vi "agilent_measurement_test.vi"() -> ()   [LabVIEW 2016]
doc: "This VI shows how to do a logarithmic frequency sweep, and query the data from the PNA."
uses:
  <instrlib>/Keysight PNA Series/Keysight PNA Series.lvlib
panel:
  in  "Sweep Points (201)":i32=201
  out "Data":dbl[](graph)
  in  "Stop Frequency (1E+10 Hz)":dbl=6000000000.0
  in  "Start Frequency (1E+6 Hz)":dbl=1000000000.0
  in  "Measurement Name (MyMeas)":string="MyMeas"
  in  "Measurement Parameters (S22)":string="S22"
  in  "Channel (1)":i32=1
  in  "VISA resource name":refnum<visa-resource-name>="vna"
  # "(c) 2017 National Instruments.  ALL RIGHTS RESERVED."
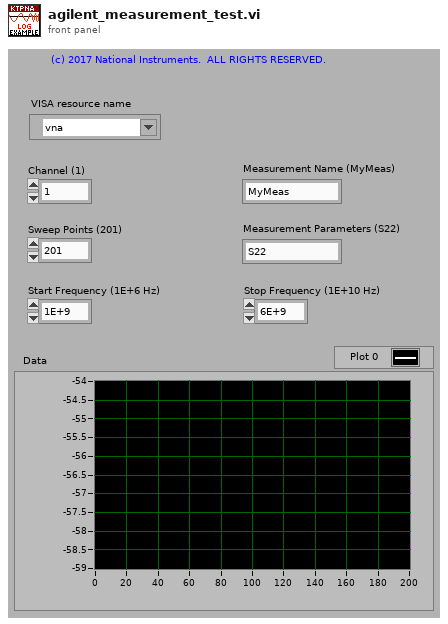
[diagram p1: front panel]
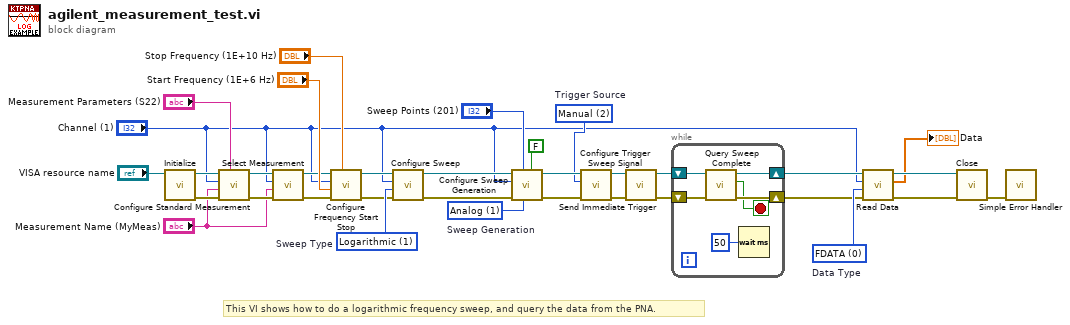
[diagram p0: block diagram]
diagram:
  w4 = 2 items=["Immediate", "External", "Manual"]  # Trigger Source
  w13 = 1 items=["Stepped", "Analog"]  # Sweep Generation
  w20 = 0 items=["FDATA", "RDATA", "SDATA", "FMEM", "SMEM", "SDIV"]  # Data Type
  w26 = 1 items=["Linear", "Logarithmic", "Power", "CW", "Segment", "Phase"]  # Sweep Type
  # "This VI shows how to do a logarithmic frequency sweep, and query the data from the PNA."
  n1 = call <instrlib>:"Initialize.vi"("VISA resource name"="VISA resource name") -> ("error out"=w32:errorcluster, "VISA resource name out"=w30:refnum<visa-resource-name>)  [unwired: 9 in]
  n2 = call <instrlib>:"Configure Standard Measurement.vi"("Measurement Parameters (S11)"="Measurement Parameters (S22)", "error in (no error)"=w32, "Measurement Name (CH1_S11_1)"="Measurement Name (MyMeas)", "Channel (1)"="Channel (1)", "VISA resource name"=w30) -> ("error out"=w31:errorcluster, "VISA resource name out"=w29:refnum<visa-resource-name>)  [unwired: 5 in]
  n3 = call <instrlib>:"Select Measurement.vi"("error in (no error)"=w31, "Measurement Name (CH1_S11_1)"="Measurement Name (MyMeas)", "Channel (1)"="Channel (1)", "VISA resource name"=w29) -> ("error out"=w10:errorcluster, "VISA resource name out"=w11:refnum<visa-resource-name>)  [unwired: 6 in]
  n4 = call <instrlib>:"Configure Frequency Start Stop.vi"("Stop Frequency (2E+6 Hz)"="Stop Frequency (1E+10 Hz)", "error in (no error)"=w10, "Start Frequency (1E+6 Hz)"="Start Frequency (1E+6 Hz)", "Channel (1)"="Channel (1)", "VISA resource name"=w11) -> ("error out"=w9:errorcluster, "VISA resource name out"=w12:refnum<visa-resource-name>)  [unwired: 5 in]
  n5 = call <instrlib>:"Configure Sweep.vi"("error in (no error)"=w9, "Sweep Type (0: Linear)"=w26, "Channel (1)"="Channel (1)", "VISA resource name"=w12) -> ("error out"=w19:errorcluster, "VISA resource name out"=w18:refnum<visa-resource-name>)  [unwired: 6 in]
  n6 = call <instrlib>:"Configure Sweep Generation.vi"("Auto Sweep or Dwell Time (T: Enable)"=FALSE ("Enable Auto Sweep/Dwell Time (T: Enable)"), "Sweep Generation (1: Analog)"=w13, "Sweep Points (201)"="Sweep Points (201)", "error in (no error)"=w19, "Channel (1)"="Channel (1)", "VISA resource name"=w18) -> ("error out"=w8:errorcluster, "VISA resource name out"=w6:refnum<visa-resource-name>)  [unwired: 4 in]
  n7 = call <instrlib>:"Configure Trigger Sweep Signal.vi"("error in (no error)"=w8, "Trigger Source (0: Immediate)"=w4, "VISA resource name"=w6) -> ("error out"=w3:errorcluster, "VISA resource name out"=w2:refnum<visa-resource-name>)  [unwired: 7 in]
  n8 = call <instrlib>:"Send Immediate Trigger.vi"("error in (no error)"=w3, "VISA resource name"=w2) -> ("error out"=w7:errorcluster, "VISA resource name out"=w5:refnum<visa-resource-name>)  [unwired: 8 in]
  n9 = while {
    shift-right: [w39] -> w15
    shift-left: w7 -> [w40]
    shift-right: [w36] -> w14
    shift-left: w5 -> [w37]
    stop <- w38 stop-if-true
    n10 = call <instrlib>:"Query Sweep Complete.vi"("error in (no error)"=w40, "VISA resource name"=w37) -> ("error out"=w39:errorcluster, "Sweep Complete"=w38:bool, "VISA resource name out"=w36:refnum<visa-resource-name>)  [unwired: 7 in]
    n11 = Wait (ms)(milliseconds to wait=u32 50) -> ()  [unwired: 1 out]
  }
  n12 = call <instrlib>:"Read Data.vi"("error in (no error)"=w15, "Data Type (0: FDATA)"=w20, "Channel (1)"="Channel (1)", "VISA resource name"=w14) -> ("error out"=w23:errorcluster, "Data"=→"Data":dbl[], "VISA resource name out"=w22:refnum<visa-resource-name>)  [unwired: 5 in]
  n13 = call <instrlib>:"Close.vi"("error in (no error)"=w23, "VISA resource name"=w22) -> ("error out"=w33:errorcluster)  [unwired: 9 in]
  n14 = call <vilib>:"Simple Error Handler.vi"("error in (no error)"=w33) -> ()  [unwired: 4 in, 5 out]
